vi "RLC_open.vi"(11 "Path":path=path "H:/CDH/CDH_control/python_CDH") -> (2 "Boolean":bool, 3 "String 2":string)   [LabVIEW 2011]
panel:
  out "Numeric":i32
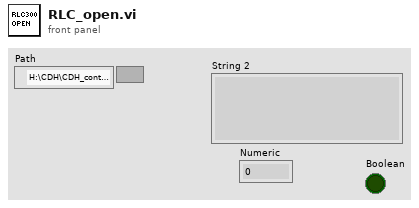
[diagram p1: front panel]
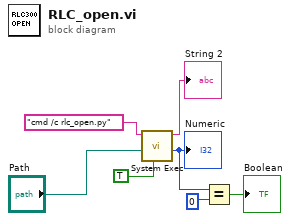
[diagram p0: block diagram]
diagram:
  n1 = call <vilib>:"System Exec.vi"("run minimized? (F)"=TRUE, "working directory"="Path", "command line"="cmd /c rlc_open.py" ("String")) -> ("return code"=w2:i32, "standard output"=→"String 2":string)  [unwired: 5 in, 2 out]
  "Numeric" <- w2
  n2 = Equal?(x=w2, y=0) -> (x = y?=→"Boolean":bool)
